vi "GpibQuery.vi"(6 "Wait (ms)":i32, 7 "Command":string, 8 "VISA resource name":refnum<visa-resource-name>) -> (0 "Error Code":i32, 1 "Error Status":bool, 2 "Error source":string, 4 "Return Value":string, 5 "Bytes Read":dbl)   [LabVIEW 2014]
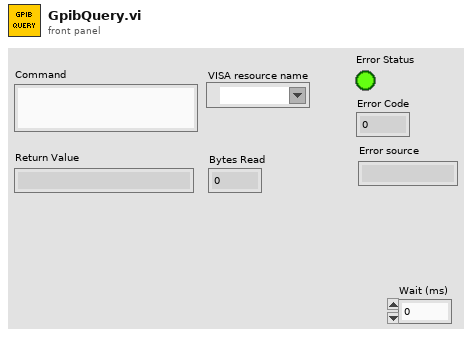
[diagram p1: front panel]
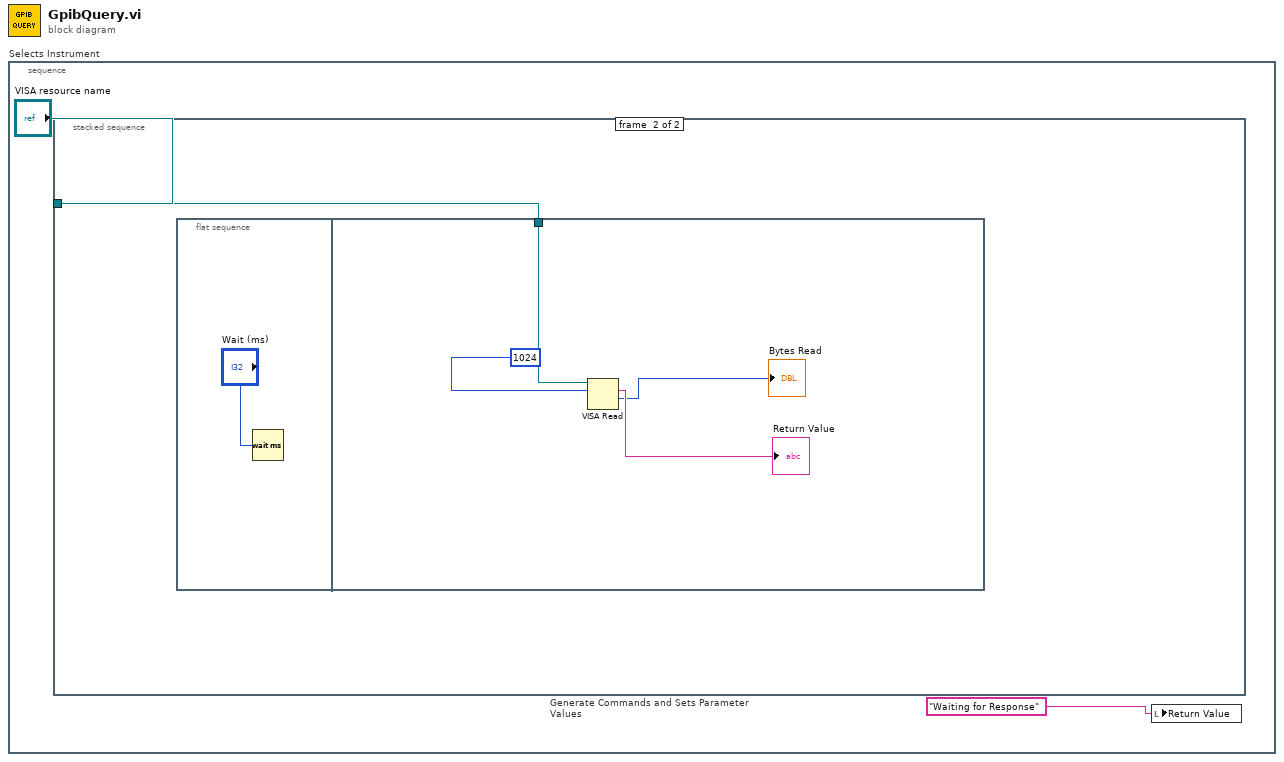
[diagram p0: block diagram]
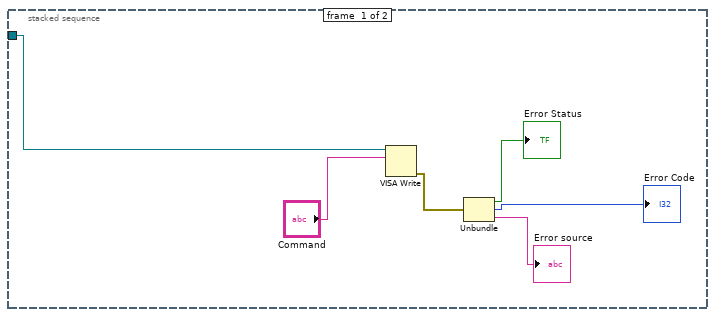
[diagram p2: hidden frame]
diagram:
  n1 = stacked-sequence "Selects Instrument" {
    frame #0 {
      n2 = stacked-sequence "Generate Commands and Sets Parameter Values" {
        tunnel: "VISA resource name" -> [w3 w9]
        frame #0 {
          n3 = VISA Write(VISA resource name=w3, write buffer="Command") -> (error out=w7:errorcluster)  [unwired: 1 in, 2 out]
          n4 = Unbundle(w7) -> ("status"=→"Error Status":bool, "code"=→"Error Code":i32, "source"=→"Error source":string)
        }
        frame #1 {
          n5 = flat-sequence {
            tunnel: w9 -> [w11]
            frame #0 {
              n6 = Wait (ms)(milliseconds to wait="Wait (ms)") -> ()  [unwired: 1 out]
            }
            frame #1 {
              n7 = VISA Read(VISA resource name=w11, byte count=1024) -> (read buffer=→"Return Value":string, return count=→"Bytes Read":u32)  [unwired: 1 in, 2 out]
            }
          }
        }
      }
      n8 = local write "Return Value"("Waiting for Response") -> ()
    }
  }
